vi "Set Dialog Position WRT 1st Open Parent.vi"(4 "error in":errorcluster, 6 "Dialog Reference":refnum<vi>, 7 "Caller Reference":refnum<vi>) -> (0 "error out":errorcluster, 2 "dialog reference out":refnum<vi>, 3 "caller reference out":refnum<vi>)   [LabVIEW 2010]
panel:
  # "This VI will center the front panel window of a VI on the open front panel of a specified caller.\nIf no caller is specified, then it will find the first caller in the call chain with an open front panel\nand center on that.  If no VI in the call chain is open, it will center itself on the screen."
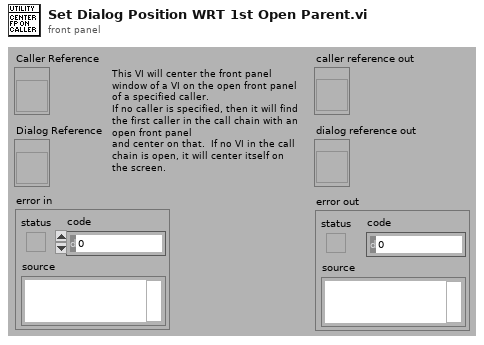
[diagram p1: front panel]
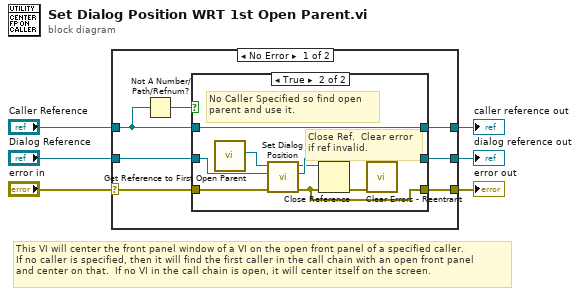
[diagram p0: block diagram]
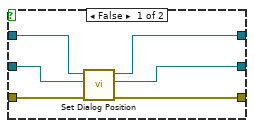
[diagram p2: hidden frame]
diagram:
  # "This VI will center the front panel window of a VI on the open front panel of a specified caller.\nIf no caller is specified, then it will find the first caller in the call chain with an open front panel\nand center on that.  If no VI in the call chain is open, it will center itself on the screen."
  n1 = case shown="No Error" "error in" {
    selector: "error in" -> [w7 w30]
    tunnel: "Dialog Reference" -> [w13 w29]
    tunnel: [w12 w30] -> w5
    tunnel: [w11 w29] -> w4
    tunnel: [w10 w28] -> w3
    tunnel: "Caller Reference" -> [w8 w28]
    frame No Error {
      n2 = Not A Number/Path/Refnum?(number/path/refnum=w8) -> (NaN/Path/Refnum?=w9:bool)
      n3 = case shown="True" w9 {
        tunnel: w13 -> [w17 w27]
        tunnel: [w18 w20] -> w12
        tunnel: w7 -> [w19 w26]
        tunnel: [w16 w25] -> w11
        tunnel: [w14 w23] -> w10
        tunnel: w8 -> [w15 w23]
        frame False {
          n4 = call "Set Dialog Position.vi"("error in (no error)"=w19, "dialog reference"=w17, "caller reference"=w15) -> ("error out"=w18:errorcluster, "dialog reference out"=w16:refnum<vi>, "caller reference out"=w14:refnum<vi>)  [unwired: 2 out]
        }
        frame True {
          # "Close Ref.  Clear error\nif ref invalid."
          # "No Caller Specified so find open\nparent and use it."
          n5 = call "Get Reference to First Open Parent.vi"() -> ("vi reference (close me!)"=w24:refnum<vi>)  [unwired: 7 out]
          n6 = call "Set Dialog Position.vi"("error in (no error)"=w26, "dialog reference"=w27, "caller reference"=w24) -> ("error out"=w20:errorcluster, "dialog reference out"=w25:refnum<vi>, "caller reference out"=w21:refnum<vi>)  [unwired: 2 out]
          n7 = Close Reference(reference=w21, error in (no error)=w20) -> (error out=w22:errorcluster)
          n8 = call "Clear Errors - Reentrant.vi"("error in (no error)"=w22) -> ()  [unwired: 7 out]
        }
      }
    }
    frame Error {
    }
  }
  "error out" <- w5
  "dialog reference out" <- w4
  "caller reference out" <- w3
